vi "Relative Path.vi"(10 "Child":path, 11 "Parent":path) -> (3 "Child Relative Path":path)   [LabVIEW 2019, in "Script.lvlib"]
doc: "Returns the relative path of the child path to the parent path.\n\nCreated by: Ryan Pacini"
uses:
  Script.lvlib
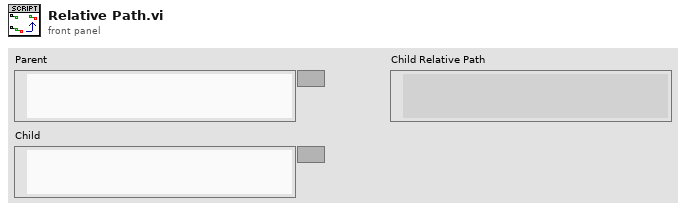
[diagram p1: front panel]
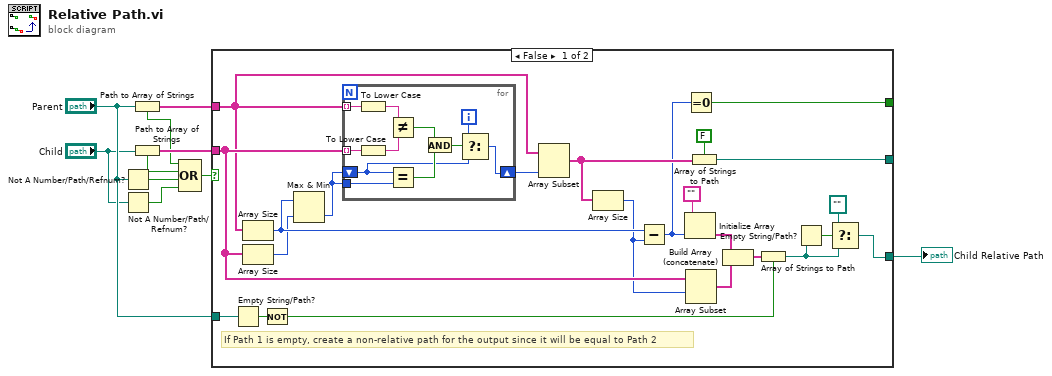
[diagram p0: block diagram]
diagram:
  n1 = Not A Number/Path/Refnum?(number/path/refnum="Parent") -> (NaN/Path/Refnum?=w2:bool)
  n2 = Not A Number/Path/Refnum?(number/path/refnum="Child") -> (NaN/Path/Refnum?=w1:bool)
  n3 = Path to Array of Strings(0:"Parent") -> (1:w3:bool, 2:w7:string[])
  n4 = Path to Array of Strings(0:"Child") -> (1:w4:bool, 2:w6:string[])
  n5 = Compound Arithmetic op=OR(w3, w4, w2, w1) -> (w5:bool)
  n6 = case shown="False" w5 {
    tunnel: w7 -> [w25 _]
    tunnel: w6 -> [w28 _]
    tunnel: [w31 _] -> _
    tunnel: [w12 _] -> w8
    tunnel: [w19 _] -> _
    tunnel: "Parent" -> [w17 _]
    frame False {
      # "If Path 1 is empty, create a non-relative path for the output since it will be equal to Path 2"
      n7 = Empty String/Path?(string/path=w17) -> (empty?=w16:bool)
      n8 = Array Size(array=w25) -> (size(s)=w24:i32)
      n9 = Array Size(array=w28) -> (size(s)=w23:i32)
      n10 = Not(x=w16) -> (.not. x?=w15:bool)
      n11 = Max & Min(x=w24, y=w23) -> (min(x,y)=w22:i32)  [unwired: 1 out]
      n12 = for {
        tunnel: w25 -> [w44] mode=indexing
        tunnel: w28 -> [w43] mode=indexing
        shift-right: [w36] -> w33
        shift-left: w22 -> [w37]
        tunnel: w22 -> [w42]
        i -> [w38]
        n13 = To Lower Case(string=w44) -> (all lower case string=w35:string)
        n14 = To Lower Case(string=w43) -> (all lower case string=w34:string)
        n15 = Not Equal?(x=w35, y=w34) -> (x != y?=w40:bool)
        n16 = Equal?(x=w37, y=w42) -> (x = y?=w41:bool)
        n17 = And(x=w40, y=w41) -> (x .and. y?=w39:bool)
        n18 = Select(t=w38, s=w39, f=w37) -> (s? t:f=w36:i32)
      }
      n19 = Array Subset(array=w25, length=w33) -> (w30:string[])  [unwired: 1 in]
      n20 = Array Size(array=w30) -> (size(s)=w21:i32)
      n21 = Subtract(x=w24, y=w21) -> (x-y=w20:i32)
      n22 = Initialize Array("", w20) -> (w29:string[])
      n23 = Equal To 0?(x=w20) -> (x = 0?=w19:bool)
      n24 = Array Subset(array=w28, index=w21) -> (w27:string[])  [unwired: 1 in]
      n25 = Array of Strings to Path(0:w30, 1:FALSE ("relative")) -> (2:w31:path)
      n26 = Build Array (concatenate)(w29, w27) -> (w26:string[])
      n27 = Array of Strings to Path(0:w26, 1:w15) -> (2:w13:path)
      n28 = Empty String/Path?(string/path=w13) -> (empty?=w14:bool)
      n29 = Select(t=path "", s=w14, f=w13) -> (s? t:f=w12:path)
    }
    frame True {
      # "If either of the paths are relative, or not a path, return error 1430."
    }
  }
  "Child Relative Path" <- w8
